vi "CSC_GetEndEffInGCS.vi"(8 "error in (no error)":errorcluster, 11 "CSC in":refnum<class "CableSerialChain.lvclass">) -> (0 "error out":errorcluster, 1 "EndEffVInGCS":dbl[](array[numeric]), 2 "EndEffInGCS":dbl[](array[numeric]) format="%#.6f", 3 "CSC out":refnum<class "CableSerialChain.lvclass">, 4 "EndEffPos":T1)   [LabVIEW 2015, in "CableSerialChain.lvclass"]
uses:
  CableSerialChain.lvclass
  Body/PointOnBody.ctl
  CableSerialChain.lvclass/CableSerialChain.ctl
  <vilib>/Analysis/BLAS.llb/gemv - General Matrix-Vector Product.vi
  <vilib>/Analysis/BLAS.llb/dgemv - General Matrix-Vector Product (DBL).vi
  <vilib>/Utility/error.llb/Error Cluster From Error Code.vi
  Body/Bodies.lvclass
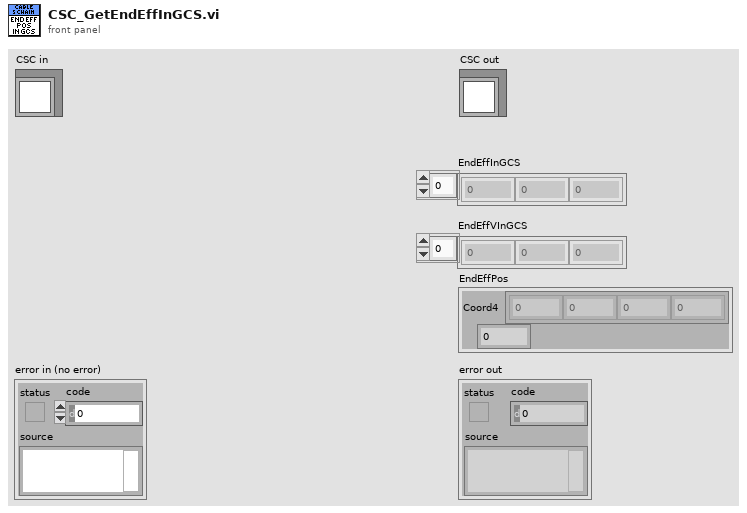
[diagram p1: front panel]
types:
  T1 = typedef "Bodies.lvclass/PointOnBody.ctl" = cluster{"Coord4":dbl[], "ID":i32}
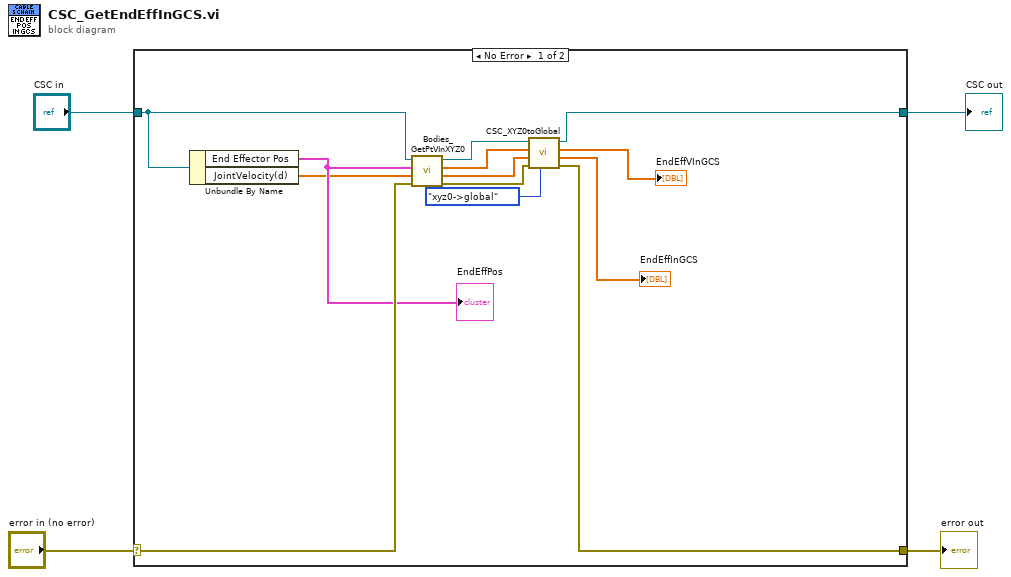
[diagram p0: block diagram]
diagram:
  n1 = case shown="No Error" "error in (no error)" {
    selector: "error in (no error)" -> [w17 w18]
    tunnel: [w9 w18] -> w3
    tunnel: [w5 w19] -> w1
    tunnel: "CSC in" -> [w7 w19]
    frame No Error {
      n2 = Unbundle By Name(w7) -> ("End Effector Pos"=w16:T1, "JointVelocity(d)"=w15:dbl[])
      "EndEffPos" <- w16
      n3 = call "Bodies_GetPtVInXYZ0.vi"("error in (no error)"=w17, "Joint V"=w15, "Point"=w16, "Bodies.lvclass"=w7) -> ("error out"=w10:errorcluster, "Pt In GCS"=w13:dbl[], "Pt V InGCS"=w14:dbl[], "Bodies.lvclass 2"=w6:refnum<class "CableSerialChain.lvclass">)  [unwired: 4 in]
      n4 = call "CSC_XYZ0toGlobal.vi"("Dir(xyz0->global)"=enum16{"global->xyz0", "xyz0->global"}."xyz0->global", "error in (no error)"=w10, "Vin"=w13, "Pin"=w14, "CSC In"=w6) -> ("error out"=w9:errorcluster, "Vout"=→"EndEffInGCS":dbl[], "Pout"=→"EndEffVInGCS":dbl[], "CSC Oout"=w5:refnum<class "CableSerialChain.lvclass">)  [unwired: 3 in]
    }
    frame Error {
    }
  }
  "error out" <- w3
  "CSC out" <- w1
